vi "choose_iphone_vi.vi"(8 "error in (no error)":errorcluster) -> (0 "error out":errorcluster, 2 "Vi to run ind":T1=enum."M1Cam" caption="Enum")   [LabVIEW 2013]
doc: "reentrant"
uses:
  VIremote.llb/VIremoteEvent.ctl
  vi picker-ajg.ctl
  VIremote.llb/VIremoteFunction.ctl
panel:
  in  "Vi to run":T1=enum."M1Cam" caption="Enum"
  in  "VIremoteEvent":T2
  # "Please choose your program to run"
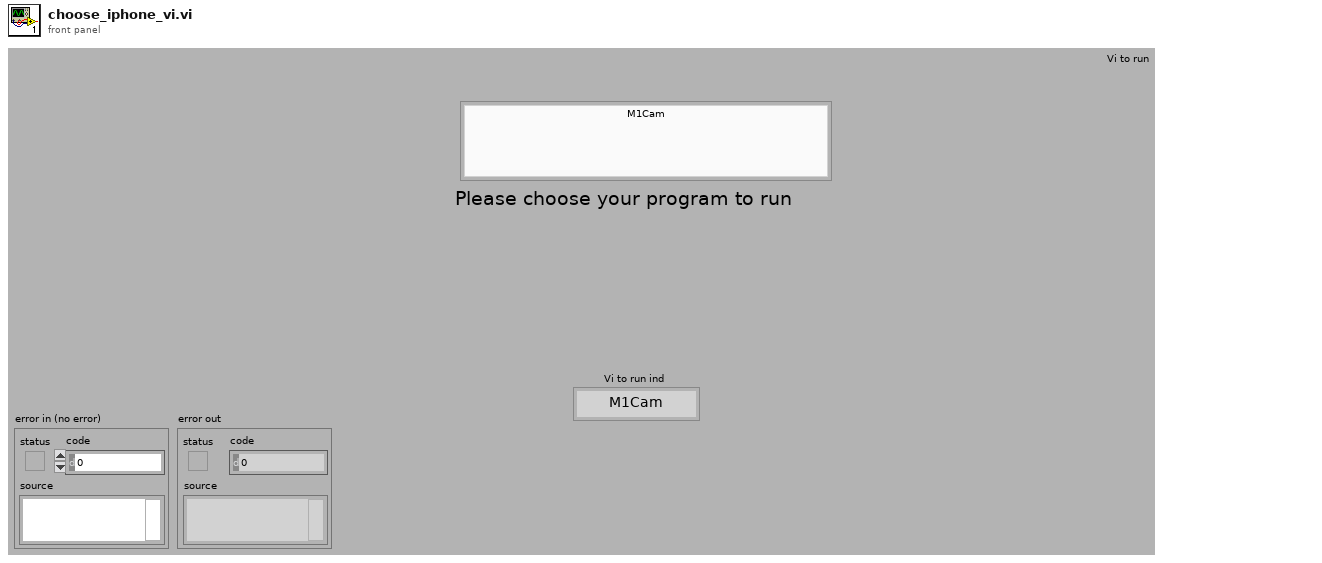
[diagram p1: front panel]
types:
  T1 = typedef "vi picker-ajg.ctl" = enum32{"Choose Something", "QUIT", "M1Cam", "M2Cam", "M4Cam", "M5Cam", "LP_Mode", "M3HPD_CCD_Near", "PhasicsHPD", "TEA_HPLBD_EnergyMeter", "LB_HPBD_EnergyMeter", "OpenHouse Demo", "demo"}
  T2 = typedef "VIremoteEvent.ctl" = enum16{"No Event", "Connection Closed", "Navigate Back", "Enter Background", "Enter Foreground", "Portrait", "Portrait Upside Down", "Landscape Left", "Landscape Right"}
  T3 = typedef "VIremoteFunction.ctl" = enum16{"Do nothing", "Stop controller", "Close this connection", "Show info panel", "Set VI to control", "Set Accelerometer freq (Hz)", "Show Alert message", "Start Sound Input", "Stop Sound Input", "Set Volume (0-100)", "Set sound output Speaker", "Set sound output Receiver", "Play Sound", "Repeat Sound", "Stop Sound", "Pause Sound", "Resume Sound", "Set panel width of caller (320 or 480)", "Set Panel Size to Portrait", "Set Panel Size to Landscape", "Set Panel Size as Current Orientation", "Allow all UI Orientations", "Send user notification", "Disable Scrolling", "Normal Scrolling", "Page Scrolling", "Set Scroll Offset", "Page Indicator Position"}
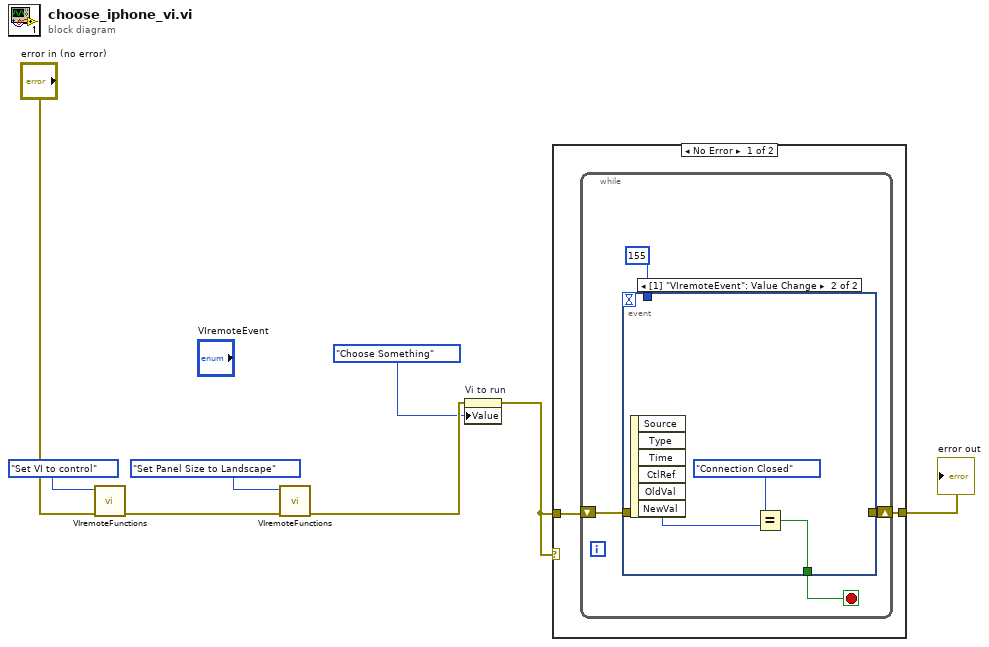
[diagram p0: block diagram]
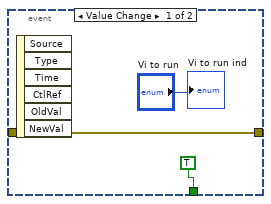
[diagram p2: hidden frame]
diagram:
  n1 = call "VIremoteFunctions.vi"("error in (no error)"="error in (no error)", "Function"=VIremoteFunction."Set VI to control") -> ("error out"=w4:errorcluster)  [unwired: 4 in, 5 out]
  n2 = call "VIremoteFunctions.vi"("error in (no error)"=w4, "Function"=VIremoteFunction."Set Panel Size to Landscape") -> ("error out"=w3:errorcluster)  [unwired: 4 in, 5 out]
  n3 = property on="Vi to run" class="Enum (strict)"(error in=w3, "Value"=vi_picker-ajg."Choose Something" ("Vi to run")) -> (error out=w2:errorcluster)  [unwired: 1 in, 1 out]
  n4 = case shown="No Error" w2 {
    tunnel: w2 -> [w10 w21]
    tunnel: [w9 w21] -> w5
    frame No Error {
      n5 = while {
        shift-right: [w12] -> w9
        shift-left: w10 -> [w13]
        stop <- w14 stop-if-true
        n6 = event shown="[1] \"VIremoteEvent\": Value Change" {
          selector: _ -> [_ _]
          dyn-events: _ -> [_ _]
          timeout: _ -> [_ _]
          tunnel: [TRUE w18] -> w14
          tunnel: w13 -> [w16 _]
          tunnel: [w16 _] -> w12
          tunnel: u32 155 ("milliseconds to wait") -> [_ _]
          event Value Change {
            n7 = event-data() -> ()  [unwired: 7 out]
            "Vi to run ind" <- "Vi to run"
          }
          event Value Change {
            n8 = event-data() -> ("NewVal"=w19:T2)  [unwired: 6 out]
            n9 = Equal?(x=VIremoteEvent."Connection Closed" ("VIremoteEvent"), y=w19) -> (x = y?=w18:bool)
          }
        }
      }
    }
    frame Error {
    }
  }
  "error out" <- w5
